vi "Practica4.vi"() -> ()   [LabVIEW 2017]
uses:
  PAGINA PRINCIPAL.ctl
panel:
  out "Sal.1":dbl
  in  "Ent.1":T1 min=0.0 max=100.0 step=0.01
  out "Tiempo transcurrido (s)":dbl
  out "Inicio":bool
  out "Fin":bool
  in  "Iniciar":bool
  in  "Calcular":bool
  # "Práctica 4: Tratamiento Térmico\n\nOBJETIVO: Estudiar los diferentes tratamientos térmicos y \ncomprender los efectos que tieneel porcentaje de carbono \nen el enfriamiento sobre las propiedades mecáncias de los \naceros."
  # "Ingrese Sección\nTransversal (mm)"
  # "Tiempo en el\nHorno (min)"
  # "LABORATORIO DE MATERIALES"
  # "LABORATORIO DE MATERIALES"
  # "OFF"
  # "ON"
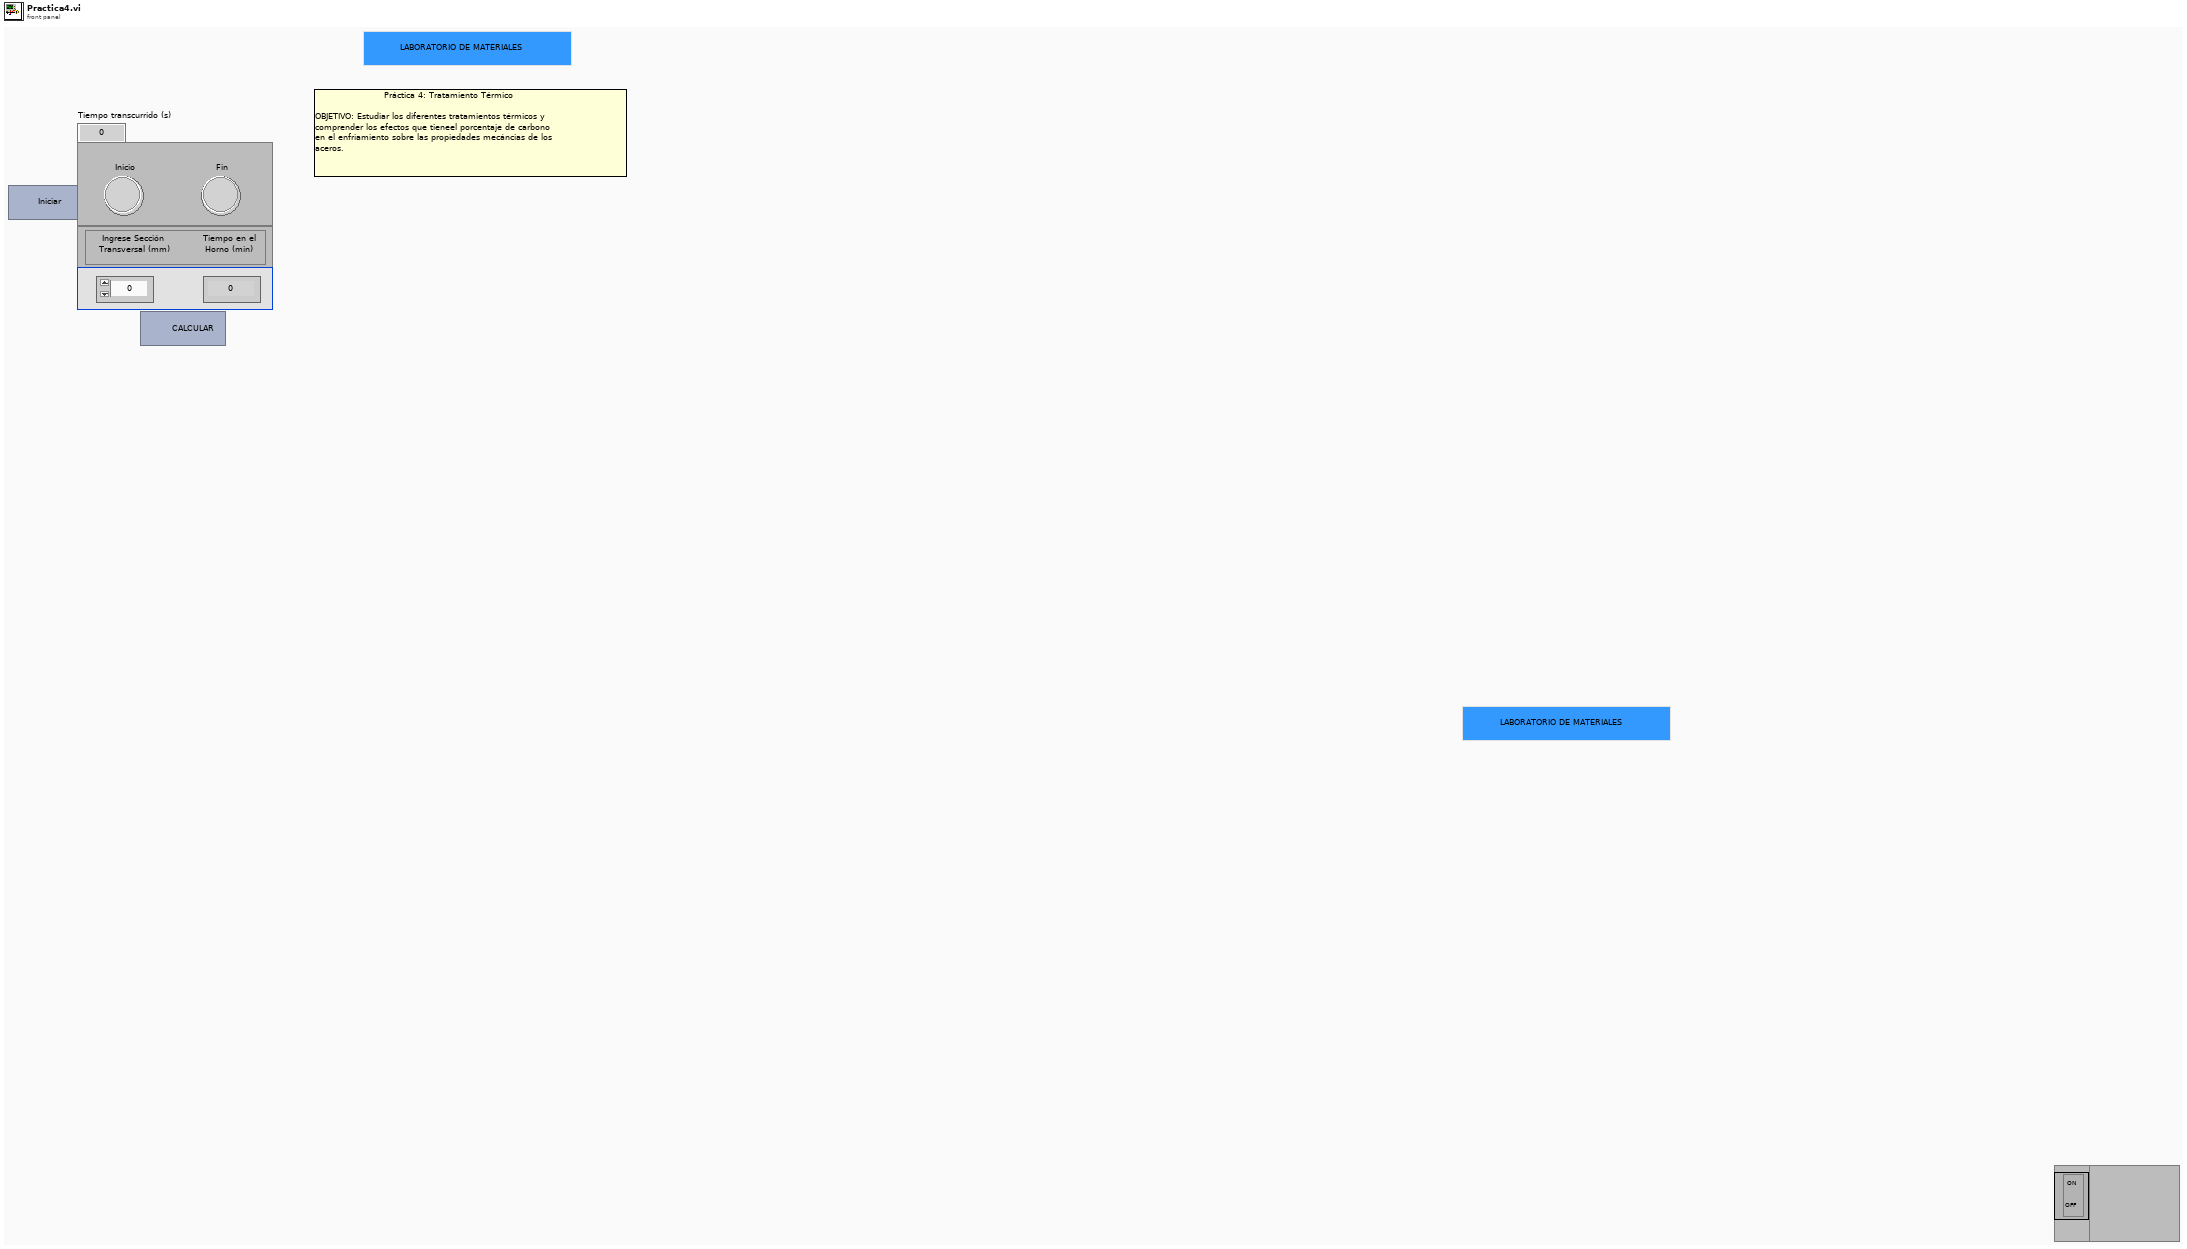
[diagram p1: front panel]
types:
  T1 = typedef "PAGINA PRINCIPAL.ctl" = dbl
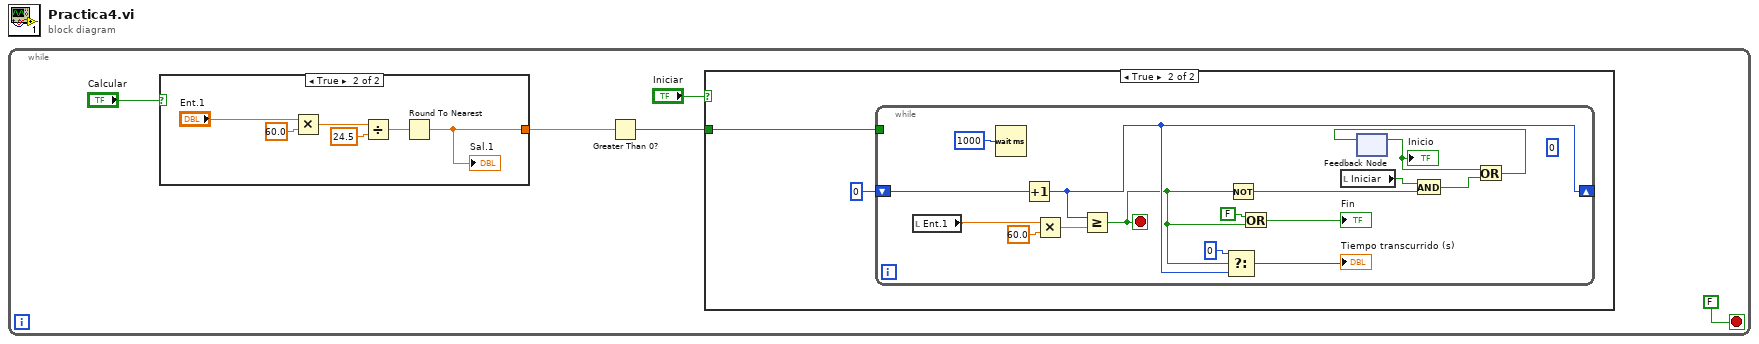
[diagram p0: block diagram]
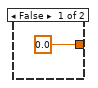
[diagram p2: hidden frame]
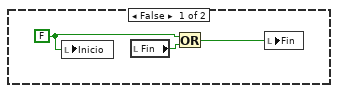
[diagram p3: hidden frame]
diagram:
  n1 = while {
    stop <- FALSE ("stop") stop-if-true
    n2 = case shown="True" "Calcular" {
      tunnel: [0.0 w7] -> w3
      frame False {
      }
      frame True {
        n3 = Multiply(x="Ent.1", y=60.0) -> (x*y=w11:T1)
        n4 = Divide(x=w11, y=24.5) -> (x/y=w9:T1)
        n5 = Round To Nearest(number=w9) -> (nearest integer value=w7:T1)
        "Sal.1" <- w7
      }
    }
    n6 = Greater Than 0?(x=w3) -> (x > 0?=w5:bool)
    n7 = case shown="True" "Iniciar" {
      tunnel: w5 -> [_ w16]
      frame False {
        w15 = FALSE ("Finalizado")
        n8 = local write "Inicio"(w15) -> ()
        n9 = local read "Fin"() -> (w13:bool)
        n10 = Or(x=w15, y=w13) -> (x .or. y?=w14:bool)
        n11 = local write "Fin"(w14) -> ()
      }
      frame True {
        n12 = while {
          shift-right: [w29] -> _
          shift-left: 0 -> [w32]
          tunnel: w16 -> [_]
          stop <- w25 stop-if-true
          (unwired) 0 ("t")
          n13 = local read "Ent.1"() -> (w18:T1)
          n14 = Wait (ms)(milliseconds to wait=u32 1000) -> ()  [unwired: 1 out]
          n15 = Increment(x=w32) -> (x+1=w29:i32)
          n16 = Multiply(x=w18, y=60.0) -> (x*y=w27:T1)
          n17 = Greater Or Equal?(x=w29, y=w27) -> (x >= y?=w25:bool)
          n18 = Select(t=0, s=w25, f=w29) -> (s? t:f=→"Tiempo transcurrido (s)":i32)
          n19 = Not(x=w25) -> (.not. x?=w26:bool)
          n20 = Or(x=FALSE ("y"), y=w25) -> (x .or. y?=→"Fin":bool)
          n21 = local read "Iniciar"() -> (w22:bool)
          n22 = feedback #1() -> (w19:bool)  [unwired: 1 in]
          "Inicio" <- w19
          n23 = And(x=w22, y=w26) -> (x .and. y?=w21:bool)
          n24 = Or(x=w19, y=w21) -> (x .or. y?=w20:bool)
          n25 = feedback-in #1(w20) -> ()
        }
      }
    }
  }
